vi "Iniltialize.vi"(8 "error in (no error)":errorcluster, 11 "Setup File in":refnum<class "Setup File.lvclass">) -> (0 "error out":errorcluster, 3 "Setup File out":refnum<class "Setup File.lvclass">)   [LabVIEW 2018, in "Setup File.lvclass"]
uses:
  Setup File.lvclass
  Setup File.lvclass/Setup File.ctl
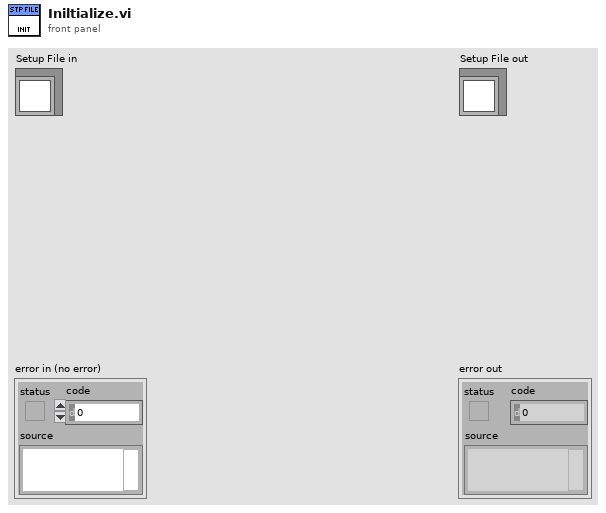
[diagram p1: front panel]
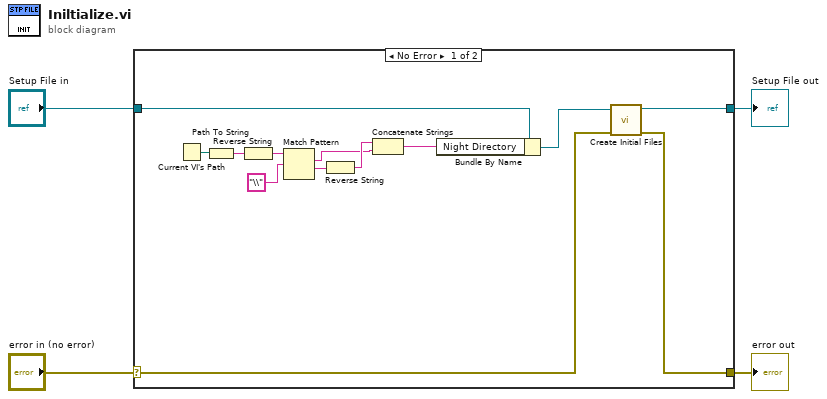
[diagram p0: block diagram]
diagram:
  n1 = case shown="No Error" "error in (no error)" {
    selector: "error in (no error)" -> [w6 w19]
    tunnel: [w5 w19] -> w3
    tunnel: [w7 w18] -> w1
    tunnel: "Setup File in" -> [w10 w18]
    frame No Error {
      n2 = Current VI's Path() -> (path=w17:path)
      n3 = Path To String(path=w17) -> (string=w16:string)
      n4 = Reverse String(1:w16) -> (0:w15:string)
      n5 = Match Pattern(string=w15, regular expression="\\") -> (match substring=w11:string, after substring=w13:string)  [unwired: 1 in, 2 out]
      n6 = Reverse String(1:w13) -> (0:w12:string)
      n7 = Concatenate Strings(w12, w11) -> (w9:string)
      n8 = Bundle By Name(cluster=w10, "Night Directory"=w9) -> (w8:refnum<class "Setup File.lvclass">)
      n9 = call "Create Initial Files.vi"("error in (no error)"=w6, "Setup File in"=w8) -> ("error out"=w5:errorcluster, "Setup File out"=w7:refnum<class "Setup File.lvclass">)  [unwired: 8 in]
    }
    frame Error {
    }
  }
  "error out" <- w3
  "Setup File out" <- w1
